vi "Ref Est.vi"(8 "IA Judge":T3) -> (0 "ref out":cluster{dbl[], "command\nenum":T1})   [LabVIEW 2016]
uses:
  Core/IA Judge.ctl
  Command Enum.ctl
panel:
  out "command":T2(ring)
  in  "command":string="Halt"
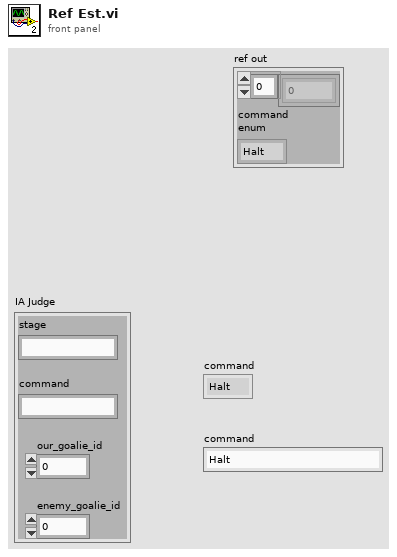
[diagram p1: front panel]
types:
  T1 = typedef "Command Enum.ctl" = enum16{"Halt", "Stop", "Force Start", "PKA Normal Start", "Prepare Kickoff Ally", "PKE Normal Start", "Prepare Kickoff Enemy", "Prepare Penalty Ally", "Prepare Penalty Enemy", "Direct Free Enemy", "Direct Free Ally", "Indirect Free Enemy", "Indirect Free Ally", "Timeout Enemy", "Timeout Ally", "Goal Enemy", "Goal Ally", "Ball Placement Enemy", "Ball Placement Ally", "None"}
  T2 = enum16{"Halt", "Stop", "Force Start", "PKA Normal Start", "Prepare Kickoff Ally", "PKE Normal Start", "Prepare Kickoff Enemy", "Prepare Penalty Ally", "Prepare Penalty Enemy", "Direct Free Enemy", "Direct Free Ally", "Indirect Free Enemy", "Indirect Free Ally", "Timeout Enemy", "Timeout Ally", "Goal Enemy", "Goal Ally", "Ball Placement Enemy", "Ball Placement Ally", "None"}
  T3 = typedef "IA Judge.ctl" = cluster{"stage":string, "command":string, "our_goalie_id":dbl, "enemy_goalie_id":dbl}
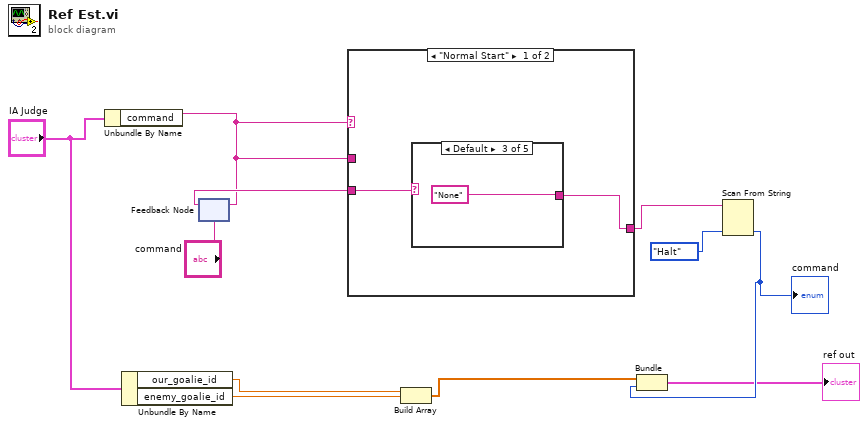
[diagram p0: block diagram]
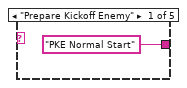
[diagram p2: hidden frame]
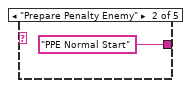
[diagram p3: hidden frame]
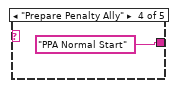
[diagram p4: hidden frame]
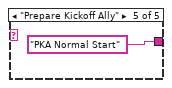
[diagram p5: hidden frame]
diagram:
  n1 = Unbundle By Name("IA Judge") -> ("command"=w7:string)
  n2 = Unbundle By Name("IA Judge") -> ("our_goalie_id"=w5:dbl, "enemy_goalie_id"=w2:dbl)
  n3 = feedback-in #1(w7) -> ()
  n4 = feedback #1("command") -> (w9:string)
  n5 = case shown="\"Normal Start\"" w7 {
    tunnel: w9 -> [w13 _]
    tunnel: [w12 w19] -> w8
    tunnel: w7 -> [_ w19]
    frame "Normal Start" {
      n6 = case shown="Default" w13 {
        tunnel: ["PKE Normal Start" "PPE Normal Start" "None" "PPA Normal Start" "PKA Normal Start"] -> w12
        frame "Prepare Kickoff Enemy" {
        }
        frame "Prepare Penalty Enemy" {
        }
        frame Default {
        }
        frame "Prepare Penalty Ally" {
        }
        frame "Prepare Kickoff Ally" {
        }
      }
    }
    frame Default {
    }
  }
  n7 = Build Array(w5, w2) -> (w4:dbl[])
  n8 = Scan From String(input string=w8, default 1=Command_Enum."Halt" ("command\nenum")) -> (output 1=w3:T1)  [unwired: 3 in, 3 out]
  "command" <- w3
  n9 = Bundle(w4, "command\nenum"=w3) -> (→"ref out":cluster{dbl[], "command\nenum":T1})  [unwired: 1 in]
